vi "wfm_feature calc_data.vi"(5 "mouse up pos":cluster{"X":dbl, "Y":dbl}, 7 "mouse down pos":cluster{"X":dbl, "Y":dbl}, 8 "error in (no error)":errorcluster, 11 "wfm_feature in":refnum<class "wfm_feature.lvclass">) -> (0 "error out":errorcluster, 1 "feature cluster":T2, 2 "fill graph param":T1, 3 "wfm_feature out":refnum<class "wfm_feature.lvclass">, 4 "valid":bool)   [LabVIEW 2018, in "wfm_feature.lvclass"]
uses:
  wfm_feature.lvclass
  subVI/mouse_state.ctl
  wfm_feature.lvclass/wfm_feature.ctl
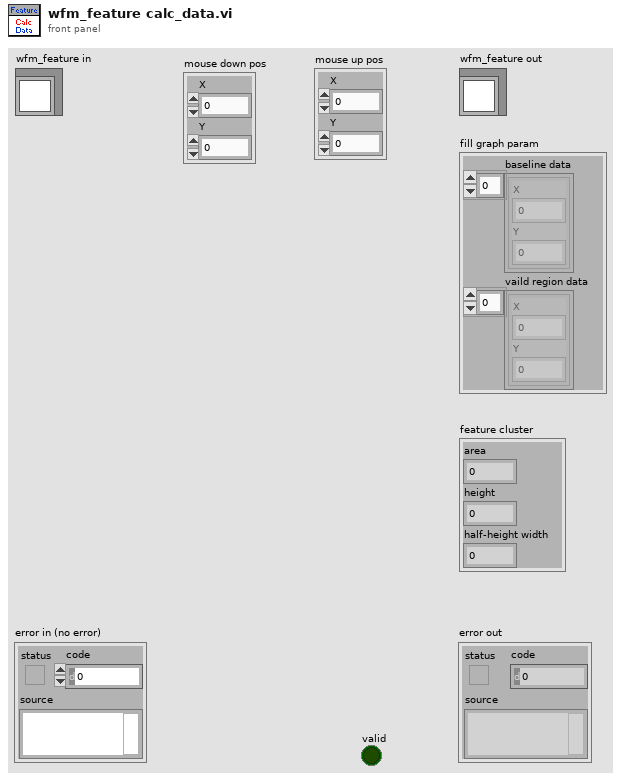
[diagram p1: front panel]
types:
  T1 = cluster{"baseline data":cluster{"X":dbl, "Y":dbl}[], "vaild region data":cluster{"X":dbl, "Y":dbl}[]}
  T2 = cluster{"area":dbl, "height":dbl, "half-height width":dbl}
  T3 = typedef "mouse_state.ctl" = enum16{"normal", "mouse down", "calc"}
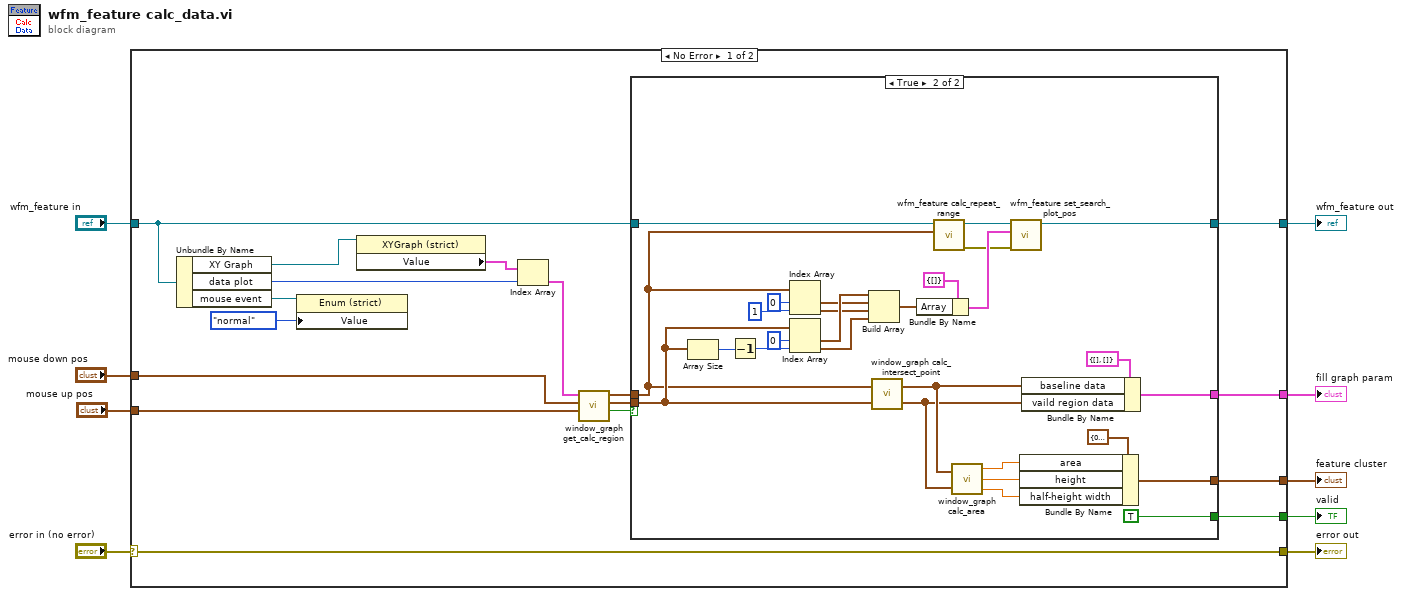
[diagram p0: block diagram]
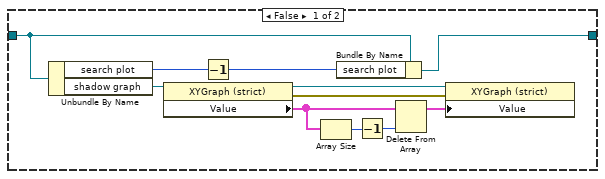
[diagram p2: hidden frame]
diagram:
  n1 = case shown="No Error" "error in (no error)" {
    selector: "error in (no error)" -> [w26 w67]
    tunnel: [w26 w67] -> w8
    tunnel: [w12 w66] -> w6
    tunnel: "wfm_feature in" -> [w13 w66]
    tunnel: "mouse down pos" -> [w23 _]
    tunnel: "mouse up pos" -> [w11 _]
    tunnel: [w22 _] -> w2
    tunnel: [w20 _] -> w3
    tunnel: [w19 _] -> w1
    frame No Error {
      n2 = Unbundle By Name(w13) -> ("XY Graph"=w18:refnum<vi>, "data plot"=w16:i32, "mouse event"=w10:refnum<vi>)
      n3 = property class="Enum (strict)"(reference=w10, "Value"=mouse_state."normal") -> ()  [unwired: 1 in, 2 out]
      n4 = property class="XYGraph (strict)"(reference=w18) -> ("Value"=w17:cluster{dbl[], sgl[]}[])  [unwired: 1 in, 2 out]
      n5 = Index Array(array=w17, index=w16) -> (element=w15:cluster{dbl[], sgl[]})
      n6 = call "window_graph get_calc_region.vi"("mouse up pos"=w11, "mouse down pos"=w23, "element"=w15) -> ("valid"=w21:bool, "region data"=w24:cluster{"X":dbl, "Y":dbl}[], "limit data"=w25:cluster{"X":dbl, "Y":dbl}[])  [unwired: 6 in]
      n7 = case shown="True" w21 {
        tunnel: w25 -> [_ w48]
        tunnel: w24 -> [_ w58]
        tunnel: [_ w52] -> w22
        tunnel: [_ TRUE] -> w20
        tunnel: [_ w60] -> w19
        tunnel: w13 -> [w27 w49]
        tunnel: [w28 w40] -> w12
        frame False {
          n8 = Unbundle By Name(w27) -> ("search plot"=w30:i32, "shadow graph"=w37:refnum<vi>)
          n9 = property class="XYGraph (strict)"(reference=w37) -> (reference out=w34:refnum<vi>, error out=w33:errorcluster, "Value"=w36:cluster{"Array":cluster{"X":dbl, "Y":dbl}[]}[])  [unwired: 1 in]
          n10 = Decrement(x=w30) -> (x-1=w29:i32)
          n11 = Array Size(array=w36) -> (size(s)=w35:i32)
          n12 = Bundle By Name(cluster=w27, "search plot"=w29) -> (w28:refnum<class "wfm_feature.lvclass">)
          n13 = Decrement(x=w35) -> (x-1=w31:i32)
          n14 = Delete From Array(array=w36, index=w31) -> (array with subset deleted=w32:cluster{"Array":cluster{"X":dbl, "Y":dbl}[]}[])  [unwired: 1 in, 1 out]
          n15 = property class="XYGraph (strict)"(reference=w34, error in=w33, "Value"=w32) -> ()  [unwired: 2 out]
        }
        frame True {
          n16 = Array Size(array=w58) -> (size(s)=w57:i32)
          n17 = Decrement(x=w57) -> (x-1=w56:i32)
          n18 = Index Array(array=w48, index #1=0 ("index"), index #2=1 ("index")) -> (element #1=w45:cluster{"X":dbl, "Y":dbl}, element #2=w44:cluster{"X":dbl, "Y":dbl})
          n19 = Index Array(array=w58, index #1=0 ("index"), index #2=w56) -> (element #1=w46:cluster{"X":dbl, "Y":dbl}, element #2=w43:cluster{"X":dbl, "Y":dbl})
          n20 = Build Array(w46, w45, w44, w43) -> (w42:cluster{"X":dbl, "Y":dbl}[])
          n21 = call "window_graph calc_intersect_point.vi"("region data"=w58, "limit data"=w48) -> ("vaild region data"=w53:cluster{"X":dbl, "Y":dbl}[], "baseline data"=w54:cluster{"X":dbl, "Y":dbl}[])
          n22 = Bundle By Name(cluster=cluster{"Array":cluster{"X":dbl, "Y":dbl}[]} {"Array"=[]} ("element"), "Array"=w42) -> (w39:cluster{"Array":cluster{"X":dbl, "Y":dbl}[]})
          n23 = call "wfm_feature calc_repeat_range.vi"("limit data"=w48, "wfm_feature in"=w49) -> ("error out"=w38:errorcluster, "wfm_feature out"=w41:refnum<class "wfm_feature.lvclass">)  [unwired: 8 in]
          n24 = call "window_graph calc_area.vi"("baseline data"=w54, "vaild region data"=w53) -> ("area"=w63:dbl, "height"=w62:dbl, "half-height width"=w61:dbl)
          n25 = call "wfm_feature set_search_plot_pos.vi"("error in (no error)"=w38, "new search plot pos"=w39, "wfm_feature in"=w41) -> ("wfm_feature out"=w40:refnum<class "wfm_feature.lvclass">)  [unwired: 7 in, 1 out]
          n26 = Bundle By Name(cluster=T2 {"area"=0.0, "height"=0.0, "half-height width"=0.0}, "area"=w63, "height"=w62, "half-height width"=w61) -> (w60:T2)
          n27 = Bundle By Name(cluster=T1 {"baseline data"=[], "vaild region data"=[]}, "baseline data"=w54, "vaild region data"=w53) -> (w52:T1)
        }
      }
    }
    frame Error {
    }
  }
  "error out" <- w8
  "wfm_feature out" <- w6
  "valid" <- w3
  "feature cluster" <- w1
  "fill graph param" <- w2
